vi "Set Trace Delay.vi"(8 "error in (no error)":errorcluster, 10 "Trace Delay ms":u32, 11 "Engine in":refnum<class "Engine.lvclass">) -> (0 "error out":errorcluster, 3 "Engine out":refnum<class "Engine.lvclass">)   [LabVIEW 2020, in "TSnax.lvlib" / "Engine.lvclass"]
uses:
  Engine.lvclass
  Engine.lvclass/Engine.ctl
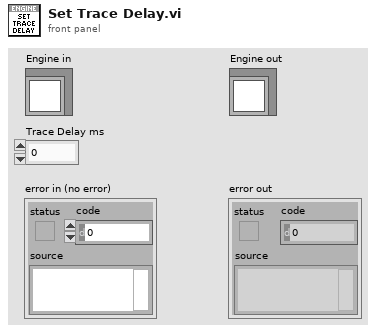
[diagram p1: front panel]
types:
  T1 = typedef "TSnax.lvlib/Engine.lvclass/Ref Data.ctl" = cluster{"Station Globals":refnum<class "PropertyObject.lvclass">, "Station Model":refnum<class "SequenceFile.lvclass">, "Trace Delay":u32}
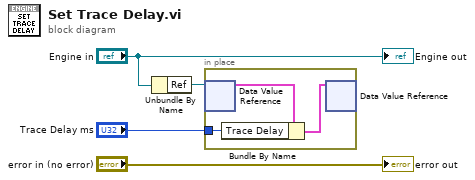
[diagram p0: block diagram]
diagram:
  n1 = Unbundle By Name("Engine in") -> ("Ref"=w3:refnum<data-value>)
  n2 = in-place {
    in-place-border: "Trace Delay ms" -> [w5]
    n3 = in-place-dvr #1(w3) -> (w7:T1)  [unwired: 1 out]
    n4 = Bundle By Name(cluster=w7, "Trace Delay"=w5) -> (w6:T1)
    n5 = in-place-dvr #1(w6) -> ()  [unwired: 2 out]
  }
  "error out" <- "error in (no error)"
  "Engine out" <- "Engine in"
